vi "Extractor pasos para montura zaber.vi"(11 "Datos Zaber":T1) -> (2 "to Zaber":T2={"Device Number"=0, "Command"=55, "Data"=0, "Response Count"=1} {"Command" items=["Echo"=55, "Home"=1, "Move Absolute"=20, "Move Relative"=21, "Move at Constant Speed"=22, "Renumber"=2, "Restore Settings"=36, "Stop"=23]})   [LabVIEW 2020]
doc: "Este vi extrae el parámetro de cuantos pasos va a moverse en función de los parámetros de la adquisición."
uses:
  <instrlib>/ZaberTSeries/Public/Utility/Request.ctl
  <instrlib>/ZaberTSeries/ZaberTSeries.lvlib
  Type Definitions/Datos Zaber.ctl
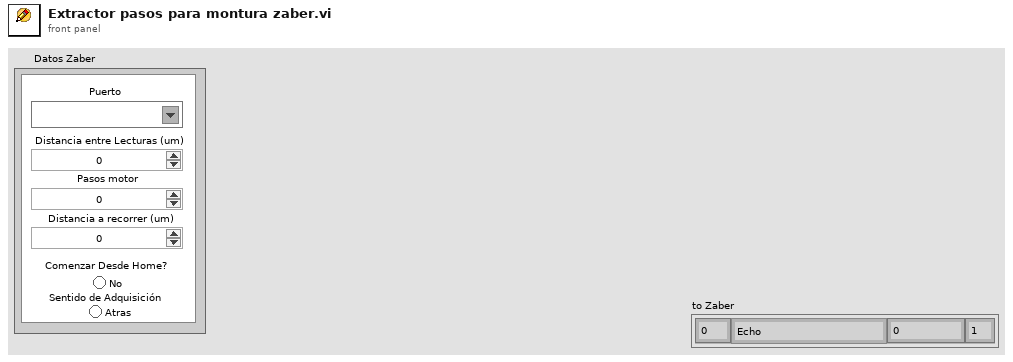
[diagram p1: front panel]
types:
  T1 = typedef "Datos Zaber.ctl" = cluster{"Sentido de Adquisición":bool, "Comenzar Desde Home?":bool, "Distancia a recorrer (um)":dbl, "Pasos motor":i32, "Distancia entre Lecturas (um)":dbl, "Puerto":refnum<visa-resource-name>}
  T2 = typedef "ZaberTSeries.lvlib/Request.ctl" = cluster{"Device Number":u8, "Command":u8, "Data":i32, "Response Count":i32}
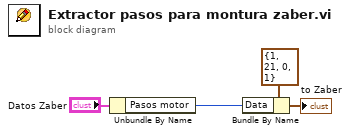
[diagram p0: block diagram]
diagram:
  n1 = Unbundle By Name("Datos Zaber") -> ("Pasos motor"=w2:i32)
  n2 = Bundle By Name(cluster=T2 {"Device Number"=1, "Command"=21, "Data"=0, "Response Count"=1} ("Request"), "Data"=w2) -> (→"to Zaber":T2)
